vi "Convert OLE Color (word).vi"(1 "color in":u32(colorbox)=16711680) -> (0 "color out":u32(colorbox)=255)   [LabVIEW 2020, in "NI_ReportGenerationToolkit.lvlib"]
doc: "Converts LabVIEW colors to or from colors used by ActiveX. All of the colors can be set using the property page for the 3D graph. Color conversion is necessary for use with ActiveX property nodes."
uses:
  <vilib>/addons/_office/NI_ReportGenerationToolkit.lvlib
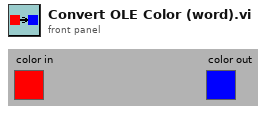
[diagram p1: front panel]
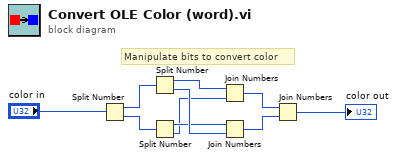
[diagram p0: block diagram]
diagram:
  # "Manipulate bits to convert color"
  n1 = Split Number(x="color in") -> (hi(x)=w4:u16, lo(x)=w3:u16)
  n2 = Split Number(x=w4) -> (hi(x)=w8:u8, lo(x)=w7:u8)
  n3 = Split Number(x=w3) -> (hi(x)=w6:u8, lo(x)=w5:u8)
  n4 = Join Numbers(hi=w8, lo=w5) -> ((hi.lo)=w1:u16)
  n5 = Join Numbers(hi=w6, lo=w7) -> ((hi.lo)=w2:u16)
  n6 = Join Numbers(hi=w1, lo=w2) -> ((hi.lo)=→"color out":u32)
